vi "Source Type.vi"(11 "User BluelinesRedlines in":refnum<class "User BluelinesRedlines.lvclass">) -> (2 "Source Type":string)   [LabVIEW 2020, in "VolatusGUIElements.lvlib" / "User BluelinesRedlines.lvclass"]
uses:
  User BluelinesRedlines.lvclass
  User BluelinesRedlines.lvclass/User BluelinesRedlines.ctl
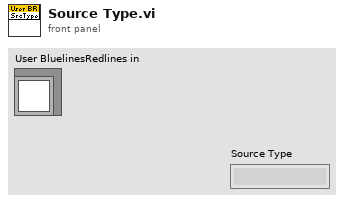
[diagram p1: front panel]
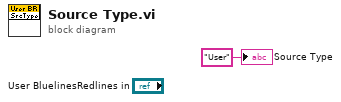
[diagram p0: block diagram]
diagram:
  "Source Type" <- "User" ("Source Type")
